vi "Merge Files.vi"(7 "Controller List":T2(array[cluster]), 8 "TemplatePath":path, 9 "CMD Step":dbl format="%#_13g", 11 "Created/ModFiles":cluster{"FilePath":path, "Save?":bool}[](array[cluster])) -> ()   [LabVIEW 2013]
uses:
  TypeDef/Controller Names.ctl
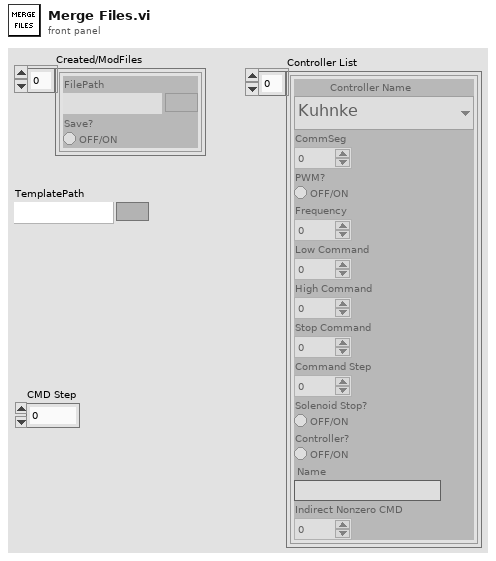
[diagram p1: front panel]
types:
  T1 = typedef "Controller Names.ctl" = enum16{"Kuhnke", "McLaren", "Helbako BLDC", "Conti", "Hella E4LMF", "Hella E4LMD", "Hella E4DCG 20mm", "Hella E4DCG 30mm", "Helbako (old)", "TI PWM", "PSA", "Hella Hyundai Gas", "Hella Hyundai Diesel", "8 Comm", "10 Comm", "8 Comm Hella FCA", "10 Comm Hella FCA", "8 Comm Omron", "10 Comm Omron", "8 Comm Nissan", "10 Comm Nissan"}
  T2 = cluster{"Controller Name":T1, "CommSeg":i32, "PWM?":bool, "Frequency":i32, "Low Command":dbl, "High Command":dbl, "Stop Command":dbl, "Command Step":dbl, "Solenoid Stop?":bool, "Controller?":bool, "Name":string, "Indirect Nonzero CMD":dbl}[]
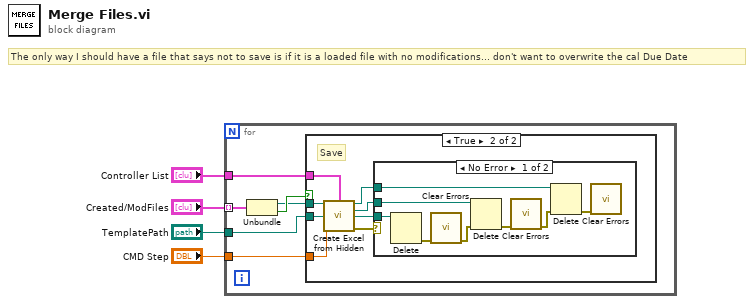
[diagram p0: block diagram]
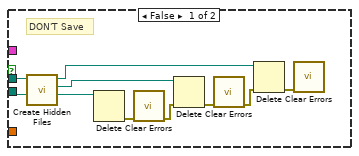
[diagram p2: hidden frame]
diagram:
  # "The only way I should have a file that says not to save is if it is a loaded file with no modifications... don't want to overwrite the cal Due Date"
  n1 = for {
    tunnel: "Created/ModFiles" -> [w10] mode=indexing
    tunnel: "TemplatePath" -> [w7]
    tunnel: "Controller List" -> [w6]
    tunnel: "CMD Step" -> [w5]
    n2 = Unbundle(w10) -> ("FilePath"=w8:path, "Save?"=w9:bool)
    n3 = case shown="True" w9 {
      tunnel: w8 -> [w20 w24]
      tunnel: w7 -> [w11 w23]
      tunnel: w6 -> [_ w22]
      tunnel: w5 -> [_ w21]
      frame False {
        # "DON'T Save"
        n4 = call "Create Hidden Files.vi"("TemplatePath"=w11, "DataFilePath"=w20) -> ("Specs Path"=w17:path, "Stats path"=w18:path, "Data Path"=w19:path)  [unwired: 7 in]
        n5 = Delete(path (use dialog)=w17) -> (error out=w16:errorcluster)  [unwired: 4 in, 2 out]
        n6 = call <vilib>:"Clear Errors.vi"("error in (no error)"=w16) -> ("error out"=w13:errorcluster)  [unwired: 6 in]
        n7 = Delete(path (use dialog)=w18, error in=w13) -> (error out=w15:errorcluster)  [unwired: 3 in, 2 out]
        n8 = call <vilib>:"Clear Errors.vi"("error in (no error)"=w15) -> ("error out"=w12:errorcluster)  [unwired: 6 in]
        n9 = Delete(path (use dialog)=w19, error in=w12) -> (error out=w14:errorcluster)  [unwired: 3 in, 2 out]
        n10 = call <vilib>:"Clear Errors.vi"("error in (no error)"=w14) -> ()  [unwired: 6 in, 1 out]
      }
      frame True {
        # "Save"
        n11 = call "Create Excel from Hidden.vi"("DataFilePath"=w24, "Controller List"=w22, "TemplatePath"=w23, "CMD Step"=w21) -> ("Stat_Path"=w25:path, "Data_Path"=w26:path, "Spec_Path"=w27:path, "Error Out"=w28:errorcluster)  [unwired: 8 in]
        n12 = case shown="No Error" w28 {
          tunnel: w27 -> [w34 _]
          tunnel: w26 -> [w35 _]
          tunnel: w25 -> [w36 _]
          frame No Error {
            n13 = Delete(path (use dialog)=w34) -> (error out=w33:errorcluster)  [unwired: 4 in, 2 out]
            n14 = call <vilib>:"Clear Errors.vi"("error in (no error)"=w33) -> ("error out"=w30:errorcluster)  [unwired: 6 in]
            n15 = Delete(path (use dialog)=w35, error in=w30) -> (error out=w32:errorcluster)  [unwired: 3 in, 2 out]
            n16 = call <vilib>:"Clear Errors.vi"("error in (no error)"=w32) -> ("error out"=w29:errorcluster)  [unwired: 6 in]
            n17 = Delete(path (use dialog)=w36, error in=w29) -> (error out=w31:errorcluster)  [unwired: 3 in, 2 out]
            n18 = call <vilib>:"Clear Errors.vi"("error in (no error)"=w31) -> ()  [unwired: 6 in, 1 out]
          }
          frame Error {
          }
        }
      }
    }
  }
